vi "Poisson Random.vi"(6 "seed":i32=-1, 7 "reset":bool, 10 "lambda":dbl=1.0, 11 "samples":i32=128) -> (0 "error":i32, 3 "Poisson random data":i32[](array[numeric]))   [LabVIEW 2017, in "NI_Gmath.lvlib"]
doc: "Generates random values from a variate X, where X describes the selected distribution type. You must manually select the polymorphic instance to use."
uses:
  <vilib>/gmath/NI_Gmath.lvlib
  <vilib>/gmath/statdist.llb/st_error_code.ctl
  <vilib>/Analysis/NI_AALBase.lvlib
panel:
  # "Poisson Random"
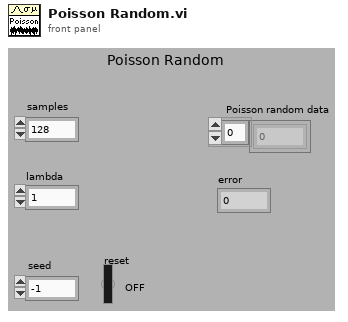
[diagram p1: front panel]
types:
  T1 = typedef "NI_Gmath.lvlib/st_error_code.ctl" = i32
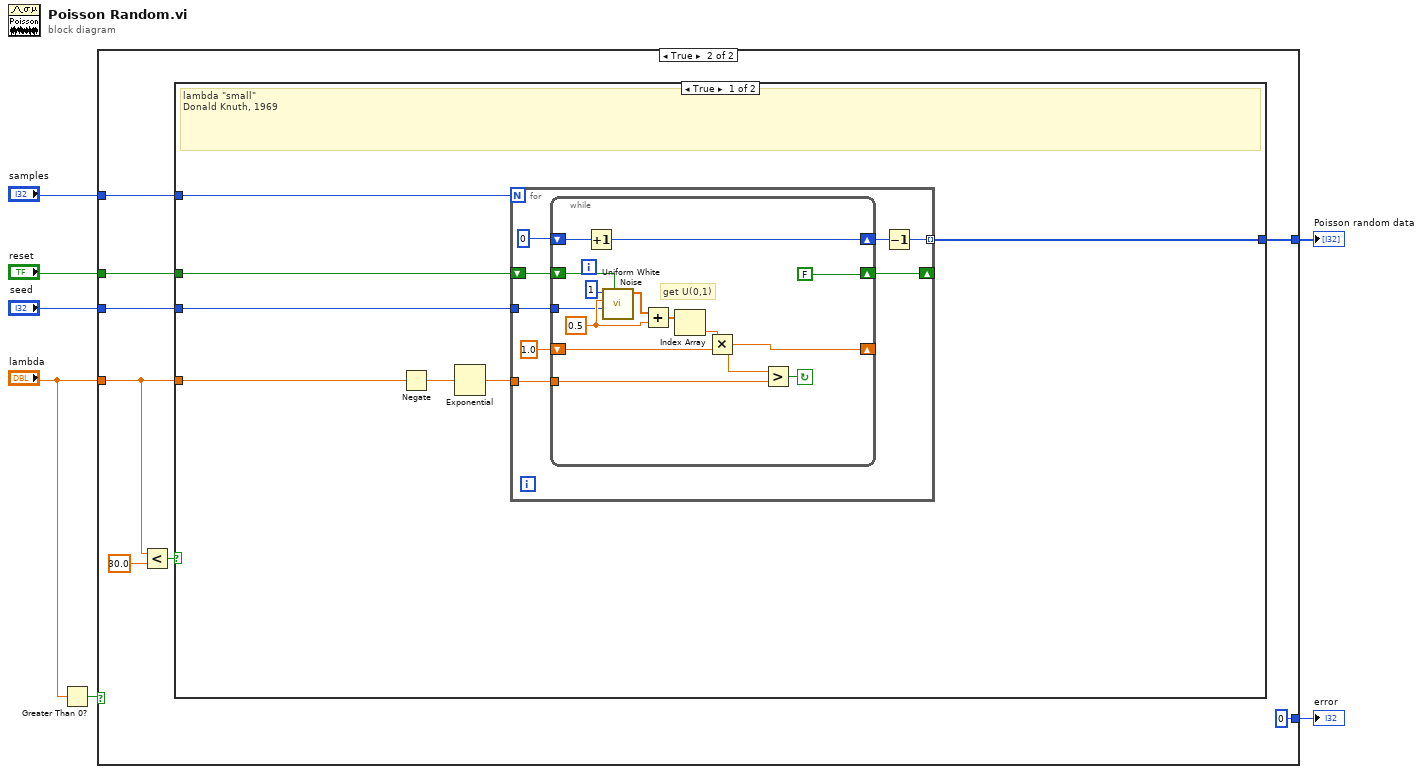
[diagram p0: block diagram]
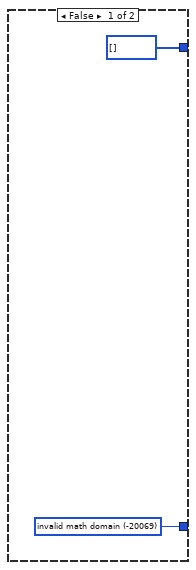
[diagram p2: hidden frame]
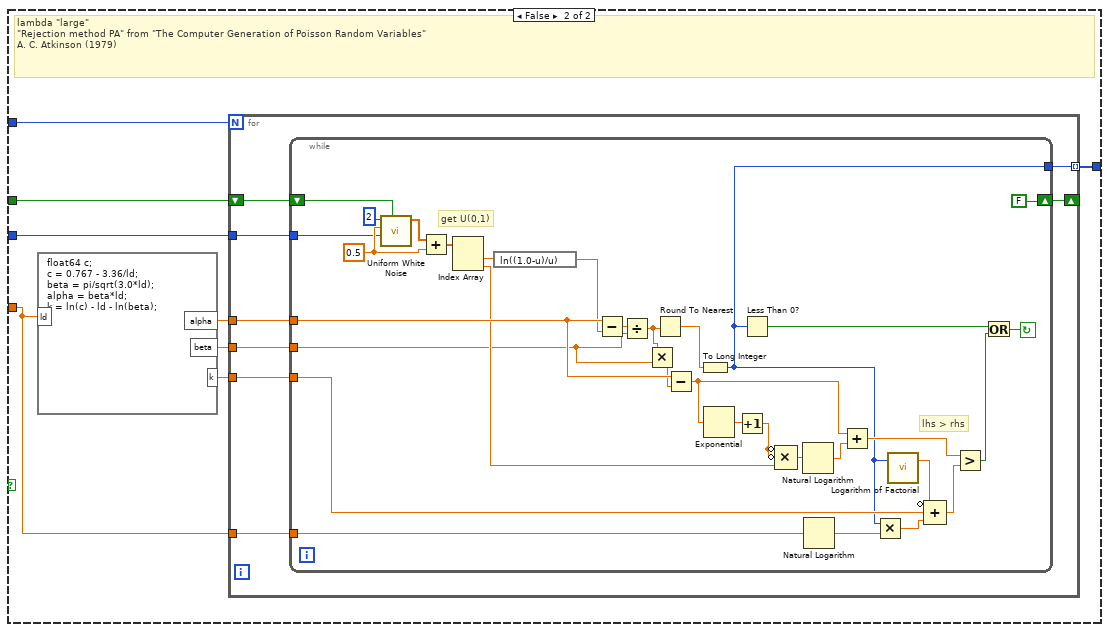
[diagram p3: hidden frame]
diagram:
  n1 = Greater Than 0?(x="lambda") -> (x > 0?=w7:bool)
  n2 = case shown="True" w7 {
    tunnel: [i32[] [] w16] -> w2
    tunnel: "lambda" -> [_ w10]
    tunnel: [w8 0 ("invalid math domain")] -> w1
    tunnel: "reset" -> [_ w15]
    tunnel: "samples" -> [_ w14]
    tunnel: "seed" -> [_ w13]
    frame False {
      w8 = T1 -20069 items=["invalid math domain"=-20069, "Fourier interpolation size m >= n"=-20070, "empty array"=-20003] ("stat interp error code")
    }
    frame True {
      n3 = Less?(x=w10, y=30.0) -> (x < y?=w12:bool)
      n4 = case shown="True" w12 {
        tunnel: w10 -> [w24 w48]
        tunnel: [w21 w47] -> w16
        tunnel: w15 -> [w20 w54]
        tunnel: w14 -> [w19 w53]
        tunnel: w13 -> [w18 w52]
        frame True {
          # "lambda \"small\"\nDonald Knuth, 1969"
          n5 = Negate(x=w24) -> (-x=w23:dbl)
          n6 = Exponential(1:w23) -> (0:w22:dbl)
          n7 = for {
            N: w19 -> [_]
            tunnel: w22 -> [w31]
            tunnel: [w29] -> w21 mode=indexing
            tunnel: w18 -> [w27]
            shift-right: [w25] -> _
            shift-left: w20 -> [w28]
            n8 = while {
              shift-right: [w45] -> w30
              shift-left: 0 -> [w46]
              shift-right: [FALSE ("reset")] -> w25
              shift-left: w28 -> [w39]
              tunnel: w31 -> [w38]
              tunnel: w27 -> [w36]
              shift-right: [w33] -> _
              shift-left: 1.0 -> [w34]
              stop <- w37 continue-if-true
              w42 = 0.5 ("amplitude")
              # "get U(0,1)"
              n9 = Increment(x=w46) -> (x+1=w45:i32)
              n10 = call <vilib>:"Uniform White Noise.vi"("initialize?"=w39, "seed"=w36, "amplitude"=w42, "samples"=1) -> ("uniform white noise"=w43:dbl[])  [unwired: 6 in, 1 out]
              n11 = Add(x=w43, y=w42) -> (x+y=w44:dbl[])
              n12 = Index Array(array=w44) -> (element=w35:dbl)  [unwired: 1 in]
              n13 = Multiply(x=w35, y=w34) -> (x*y=w33:dbl)
              n14 = Greater?(x=w33, y=w38) -> (0:w37:bool)
            }
            n15 = Decrement(x=w30) -> (x-1=w29:i32)
          }
        }
        frame False {
          # "lambda \"large\"\n\"Rejection method PA\" from \"The Computer Generation of Poisson Random Variables\"\nA. C. Atkinson (1979)"
          n16 = formula code="float64 c;\nc = 0.767 - 3.36/ld;\nbeta = pi/sqrt(3.0*ld);\nalpha = beta*ld;\nk = ln(c) - ld - ln(beta);"("ld"=w48) -> ("k"=w49:dbl, "beta"=w50:dbl, "alpha"=w51:dbl)
          n17 = for {
            N: w53 -> [_]
            tunnel: w52 -> [w61]
            tunnel: w51 -> [w60]
            tunnel: w50 -> [w59]
            tunnel: w49 -> [w58]
            tunnel: w48 -> [w57]
            tunnel: [w56] -> w47 mode=indexing
            shift-right: [w55] -> _
            shift-left: w54 -> [w62]
            n18 = while {
              shift-right: [FALSE ("reset")] -> w55
              shift-left: w62 -> [w89]
              tunnel: w61 -> [w88]
              tunnel: w60 -> [w84]
              tunnel: w59 -> [w63]
              tunnel: w58 -> [w73]
              tunnel: w57 -> [w76]
              tunnel: [w67] -> w56
              stop <- w85 continue-if-true
              w92 = 0.5 ("amplitude")
              # "lhs > rhs"
              # "get U(0,1)"
              n19 = call <vilib>:"Uniform White Noise.vi"("initialize?"=w89, "seed"=w88, "amplitude"=w92, "samples"=2) -> ("uniform white noise"=w93:dbl[])  [unwired: 6 in, 1 out]
              n20 = Add(x=w93, y=w92) -> (x+y=w94:dbl[])
              n21 = Index Array(array=w94) -> (element #1=w87:dbl, element #2=w80:dbl)  [unwired: 2 in]
              n22 = expression code="ln((1.0-u)/u)"(w87) -> (w66:dbl)
              n23 = Subtract(x=w84, y=w66) -> (x-y=w65:dbl)
              n24 = Divide(x=w65, y=w63) -> (x/y=w64:dbl)
              n25 = Multiply(x=w64, y=w63) -> (x*y=w83:dbl)
              n26 = Round To Nearest(number=w64) -> (nearest integer value=w68:dbl)
              n27 = Subtract(x=w84, y=w83) -> (x-y=w78:dbl)
              n28 = To Long Integer(number=w68) -> (32bit integer=w67:i32)
              n29 = Exponential(1:w78) -> (0:w82:dbl)
              n30 = Increment(x=w82) -> (x+1=w81:dbl)
              n31 = Less Than 0?(x=w67) -> (x < 0?=w86:bool)
              n32 = Compound Arithmetic op=MULTIPLY(invert w81, invert w81, w80) -> (w79:dbl)
              n33 = Natural Logarithm(1:w79) -> (0:w77:dbl)
              n34 = Natural Logarithm(1:w76) -> (0:w75:dbl)
              n35 = Add(x=w78, y=w77) -> (x+y=w70:dbl)
              n36 = Multiply(x=w67, y=w75) -> (x*y=w74:dbl)
              n37 = call <vilib>:"Logarithm of Factorial.vi"("n"=w67) -> ("ln(n!)"=w72:dbl)  [unwired: 2 in]
              n38 = Compound Arithmetic op=ADD(invert w72, w73, w74) -> (w71:dbl)
              n39 = Greater?(x=w70, y=w71) -> (0:w69:bool)
              n40 = Or(x=w86, y=w69) -> (x .or. y?=w85:bool)
            }
          }
        }
      }
    }
  }
  "error" <- w1
  "Poisson random data" <- w2
